vi "Default.File.ploy.Add Line to Text Log File.File Refnum.vi"(8 "error in (no error)":errorcluster, 10 "Line to Add":string, 11 "File Refnum (in)":refnum<file>) -> (0 "error out":errorcluster, 3 "File Refnum (out)":refnum<file>)   [LabVIEW 2010]
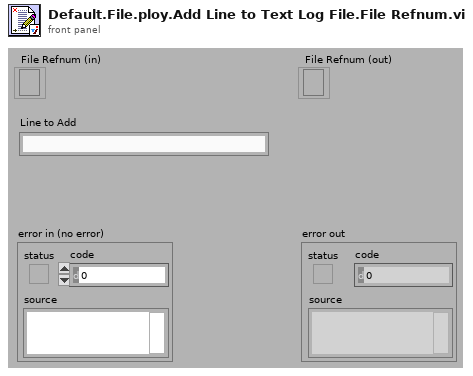
[diagram p1: front panel]
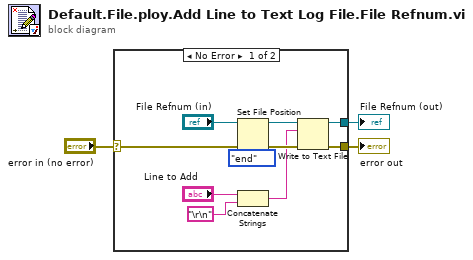
[diagram p0: block diagram]
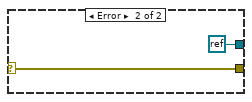
[diagram p2: hidden frame]
diagram:
  n1 = case shown="No Error" "error in (no error)" {
    selector: "error in (no error)" -> [w4 w15]
    tunnel: [w5 w15] -> w3
    tunnel: [w6 refnum<k0> refnum] -> w1
    frame No Error {
      n2 = Set File Position(refnum="File Refnum (in)", from (0:start)=enum16{"start", "end", "current"}."end", error in=w4) -> (refnum out=w11:refnum<file>, error out=w12:errorcluster)  [unwired: 1 in]
      n3 = Concatenate Strings("Line to Add", "\r\n") -> (w10:string)
      n4 = Write to Text File(file (use dialog)=w11, text=w10, error in=w12) -> (refnum out=w6:refnum<file>, error out=w5:errorcluster)  [unwired: 1 in, 1 out]
    }
    frame Error {
    }
  }
  "error out" <- w3
  "File Refnum (out)" <- w1
